vi "Read Metadata.vi"(8 "error in (no error)":errorcluster, 11 "Add Metadata Msg in":refnum<class "Add Metadata Msg.lvclass">) -> (0 "error out":errorcluster, 2 "Metadata":refnum<class "Metadata.lvclass">[](array[class]), 3 "Add Metadata Msg out":refnum<class "Add Metadata Msg.lvclass">)   [LabVIEW 2021, in "Add Metadata Msg.lvclass"]
uses:
  Add Metadata Msg.lvclass
  Add Metadata Msg.lvclass/Add Metadata Msg.ctl
  NHMFL_Core/Libraries/File/Metadata/Metadata.lvclass
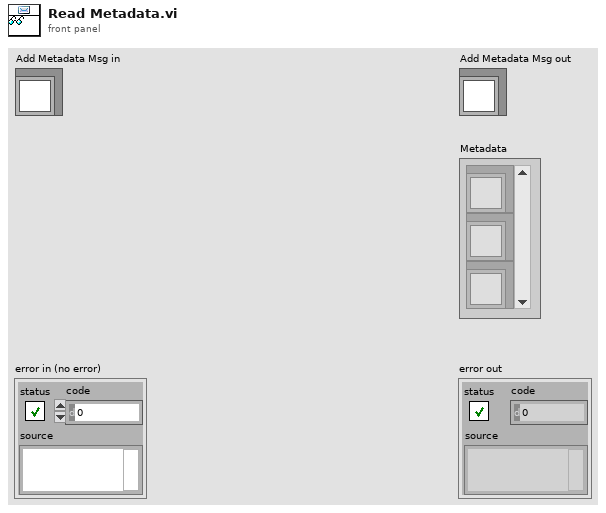
[diagram p1: front panel]
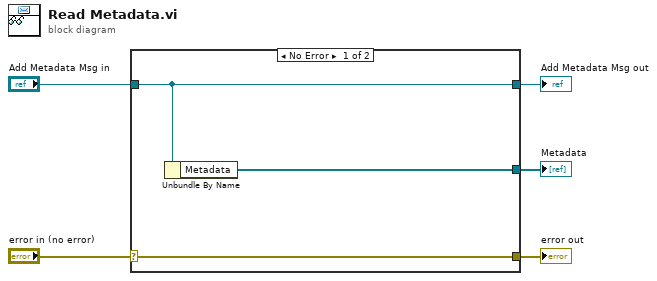
[diagram p0: block diagram]
diagram:
  n1 = case shown="No Error" "error in (no error)" {
    selector: "error in (no error)" -> [w8 w9]
    tunnel: [w8 w9] -> w4
    tunnel: [w7 w10] -> w2
    tunnel: "Add Metadata Msg in" -> [w7 w10]
    tunnel: [w6 _] -> w1
    frame No Error {
      n2 = Unbundle By Name(w7) -> ("Metadata"=w6:refnum<class "Metadata.lvclass">[])
    }
    frame Error {
    }
  }
  "error out" <- w4
  "Add Metadata Msg out" <- w2
  "Metadata" <- w1
